vi "그림전송실험클라.vi"() -> ()   [LabVIEW 2018]
panel:
  in  "파일(대화 상자 사용)":path
  out "값":path[](array[path])
  out "리스트박스":i32(listbox)
  in  "정지":bool
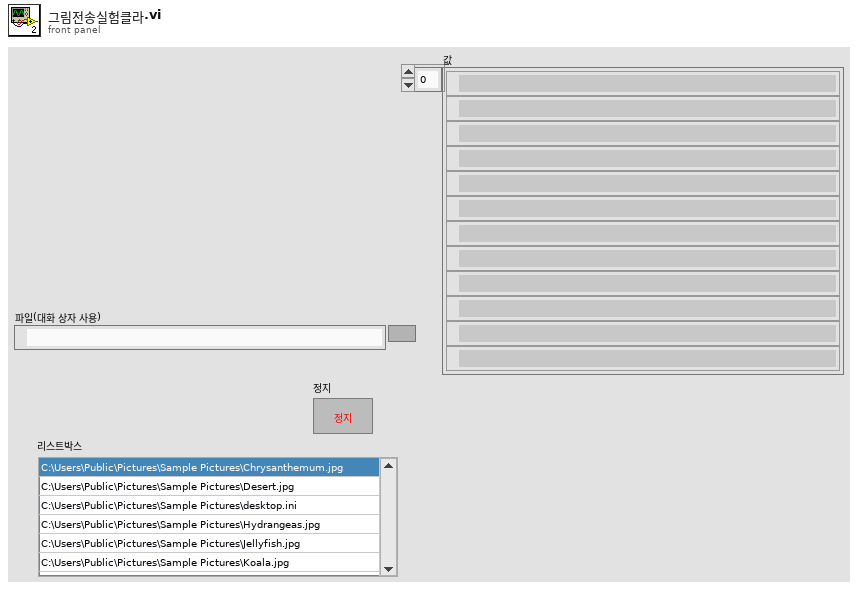
[diagram p1: front panel]
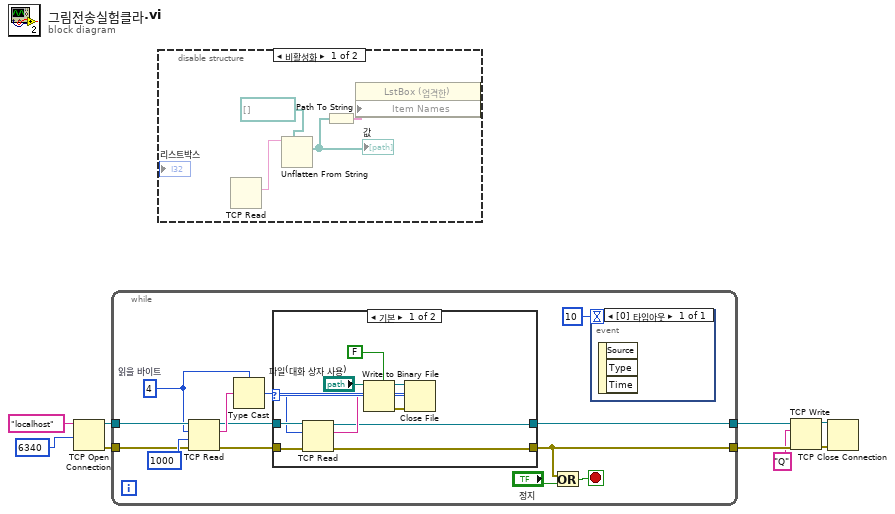
[diagram p0: block diagram]
diagram:
  n1 = TCP Open Connection(address="localhost" ("주소"), remote port or service name=u16 6340 ("포트")) -> (connection ID=w6:refnum<k5>, error out=w7:errorcluster)  [unwired: 3 in]
  n2 = while {
    tunnel: w7 -> [w21]
    tunnel: w6 -> [w20]
    tunnel: [w13] -> w4
    tunnel: [w14] -> w5
    stop <- w12 stop-if-true
    w18 = 4  # 읽을 바이트
    n3 = TCP Read(connection ID=w20, bytes to read=w18, error in (no error)=w21, 9:1000 ("타임아웃 ms (25000)")) -> (connection ID out=w15:refnum<k5>, data out=w19:string, error out=w16:errorcluster)  [unwired: 1 in]
    n4 = Type Cast(type=w18, x=w19) -> (*(type *) &x=w17:i32)
    n5 = case shown="기본" w17 {
      selector: w17 -> [w25 _]
      tunnel: w16 -> [w26 w34]
      tunnel: [w23 w34] -> w13
      tunnel: w15 -> [w27 w33]
      tunnel: [w24 w33] -> w14
      frame Default {
        n6 = TCP Read(connection ID=w27, bytes to read=w25, error in (no error)=w26) -> (connection ID out=w24:refnum<k5>, data out=w30:string, error out=w23:errorcluster)  [unwired: 2 in]
        n7 = Write to Binary File(file (use dialog)="파일(대화 상자 사용)", data=w30, 5:FALSE ("배열 또는 문자열 크기를 앞에 추가? (참)")) -> (refnum out=w28:refnum<file>, error out=w29:errorcluster)  [unwired: 3 in, 1 out]
        n8 = Close File(refnum=w28, error in=w29) -> ()  [unwired: 2 out]
      }
      frame ..0 {
      }
    }
    n9 = Or(x=w13, y="정지") -> (x .or. y?=w12:bool)
    n10 = event shown="[0] 타임아웃" {
      selector: _ -> [_]
      dyn-events: _ -> [_]
      timeout: 10 -> [_]
      event Timeout {
        n11 = event-data() -> ()  [unwired: 1 in, 3 out]
      }
    }
  }
  n12 = disable-structure shown="비활성화" {
    frame Disabled {
      n13 = TCP Read() -> (bytes to read=w37:i32, data out=w36:string)  [unwired: 4 in, 2 out]
      n14 = Unflatten From String(type=path[] [], binary string=w36) -> (value=w38:path[])  [unwired: 3 in, 2 out]
      "값" <- w38
      n15 = Path To String(path=w38) -> (string=w39:string[])
      n16 = property on="프로퍼티 노드" class="LstBox (엄격한)"("Item Names"=w39) -> ()  [unwired: 2 in, 2 out]
    }
    frame Enabled {
    }
  }
  n17 = TCP Write(connection ID=w5, data in="Q" ("데이터 입력"), error in (no error)=w4) -> (connection ID out=w2:refnum<k5>, error out=w3:errorcluster)  [unwired: 1 in, 1 out]
  n18 = TCP Close Connection(connection ID=w2, error in (no error)=w3) -> ()  [unwired: 1 in, 2 out]
